vi "Step Get By Key.vi"(8 "error in (no error)":errorcluster, 10 "ixStep":string, 11 "Connection Refnum":T2) -> (0 "error out":errorcluster, 2 "Step Record":T1, 3 "Connection Refnum":T2, 4 "Data Present":bool)   [LabVIEW 2011]
uses:
  Summitek EXT/ODBC/SQL Controls/Connection Refnum.ctl
  Step Record.ctl
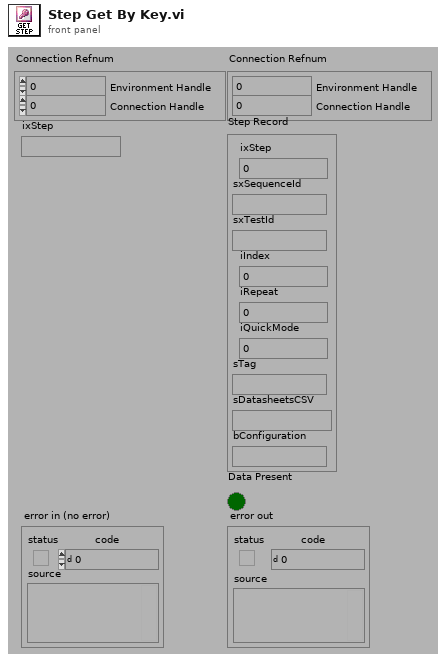
[diagram p1: front panel]
types:
  T1 = typedef "Step Record.ctl" = cluster{"ixStep":i32, "sxSequenceId":string, "sxTestId":string, "iIndex":i32, "iRepeat":i32, "iQuickMode":i32, "sTag":string, "sDatasheetsCSV":string, "bConfiguration":string}
  T2 = typedef "Connection Refnum.ctl" = cluster{"Environment Handle":i32, "Connection Handle":i32}
  T3 = typedef "Statement Refnum.ctl" = cluster{"Statement Handle":i32, "Parameter Number":u16}
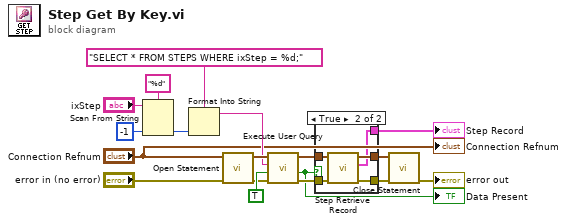
[diagram p0: block diagram]
diagram:
  n1 = Scan From String(format string="%d", input string="ixStep", default 1=-1 ("default value 1")) -> (output 1=w6:i32)  [unwired: 2 in, 3 out]
  n2 = Format Into String(format string="SELECT * FROM STEPS WHERE ixStep = %d;" ("User Query"), w6) -> (resulting string=w11:string)  [unwired: 2 in, 1 out]
  n3 = call "Open Statement.vi"("error in (no error)"="error in (no error)", "Connection Refnum"="Connection Refnum") -> ("error out"=w12:errorcluster, "Statement Refnum"=w13:T3)  [unwired: 4 out]
  n4 = call "Execute User Query.vi"("error in (no error)"=w12, "Return Data? (f)"=TRUE, "User Query"=w11, "Statement Refnum"=w13) -> ("error out"=w18:errorcluster, "Data Present?"=w10:bool, "Statement Refnum"=w17:T3)  [unwired: 1 out]
  "Data Present" <- w10
  n5 = case shown="True" w10 {
    tunnel: w18 -> [w19 w24]
    tunnel: w17 -> [w20 w25]
    tunnel: [w19 w22] -> w14
    tunnel: [w20 w23] -> w15
    tunnel: [_ w21] -> w3
    frame False {
    }
    frame True {
      n6 = call "Step Retrieve Record.vi"("error in (no error)"=w24, "Statement Refnum"=w25) -> ("error out"=w22:errorcluster, "Step"=w21:T1, "Statement Refnum"=w23:T3)  [unwired: 7 out]
    }
  }
  "Step Record" <- w3
  n7 = call "Close Statement.vi"("error in (no error)"=w14, "Statement Refnum"=w15) -> ("error out"=→"error out":errorcluster)  [unwired: 5 out]
  "Connection Refnum" <- "Connection Refnum"
